vi "Read Refrigerant File_d.vi"(6 "error in (no error)":errorcluster, 7 "Clear Memory":bool, 8 "Refprop Main Directory":path, 9 "Refrigerant File":string) -> (0 "error out":errorcluster, 2 "Mixure Cluster":T1)   [LabVIEW 2017]
doc: "Developed by:\nGreg Sussman\nProcess Automation Corp\nwww.processauto.com\n(267)685-1249"
uses:
  Mixture Composition cluster_d.ctl
panel:
  out "memory counter":i32
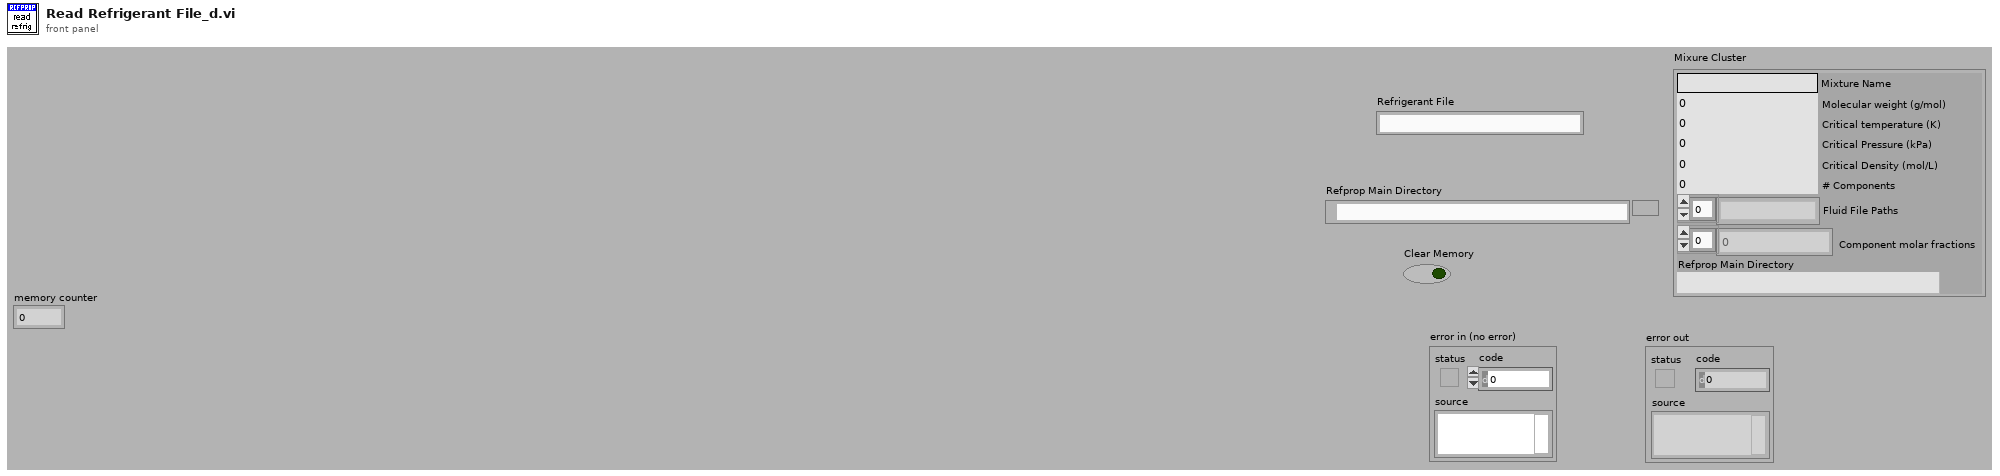
[diagram p1: front panel]
types:
  T1 = typedef "Mixture Composition cluster_d.ctl" = cluster{"Mixture Name":string, "Molecular weight (g/mol)":dbl, "Critical temperature (K)":dbl, "Critical Pressure (kPa)":dbl, "Critical Density (mol/L)":dbl, "# Components":i32, "Fluid File Paths":path[], "Component molar fractions":dbl[], "Refprop Main Directory":path}
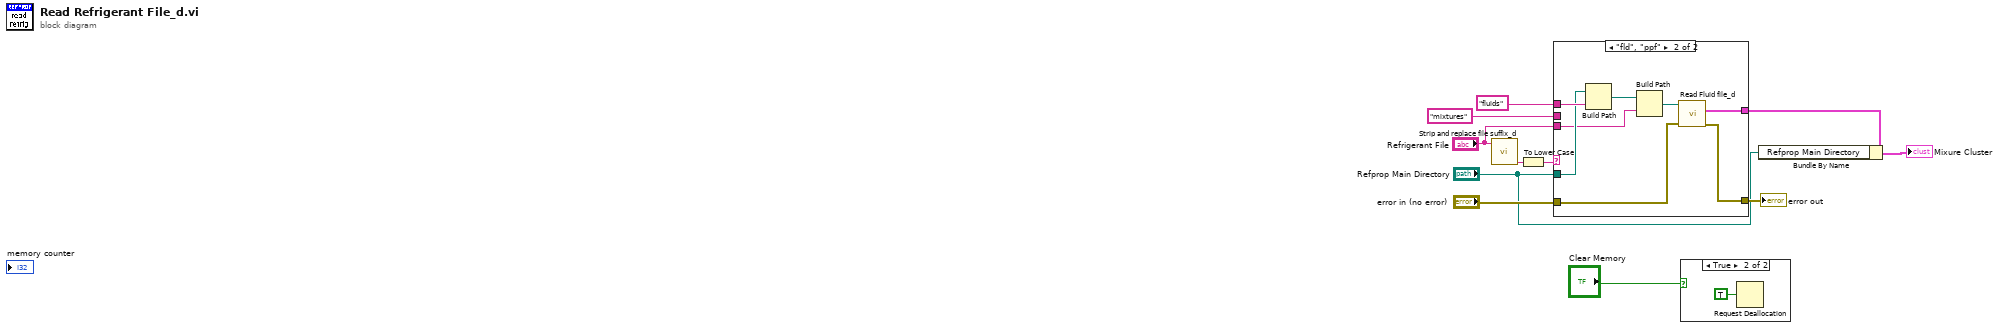
[diagram p0: block diagram]
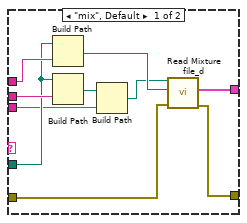
[diagram p3: hidden frame]
diagram:
  n1 = call "Strip and replace file suffix_d.vi"("File Name"="Refrigerant File") -> ("Old File Suffix OUT"=w8:string)  [unwired: 3 in, 1 out]
  n2 = To Lower Case(string=w8) -> (all lower case string=w11:string)
  n3 = case shown="\"fld\", \"ppf\"" w11 {
    tunnel: "Refprop Main Directory" -> [w15 w25]
    tunnel: [w21 w29] -> w3
    tunnel: "error in (no error)" -> [w20 w28]
    tunnel: [w19 w27] -> w9
    tunnel: "fluids" -> [w16 w26]
    tunnel: "Refrigerant File" -> [w13 w23]
    tunnel: "mixtures" -> [w18 _]
    frame "mix", Default {
      n4 = Build Path(base path=w15, name or relative path=w16) -> (appended path=w14:path)
      n5 = Build Path(base path=w15, name or relative path=w18) -> (appended path=w17:path)
      n6 = Build Path(base path=w17, name or relative path=w13) -> (appended path=w12:path)
      n7 = call "Read Mixture file_d.vi"("error in (no error)"=w20, "Dir containing fluid files"=w14, "Mixture File"=w12) -> ("error out"=w19:errorcluster, "Mixure Cluster"=w21:T1)  [unwired: 5 in]
    }
    frame "fld", "ppf" {
      n8 = Build Path(base path=w25, name or relative path=w26) -> (appended path=w24:path)
      n9 = Build Path(base path=w24, name or relative path=w23) -> (appended path=w22:path)
      n10 = call "Read Fluid file_d.vi"("error in (no error)"=w28, "Fluid File"=w22) -> ("error out"=w27:errorcluster, "Fluid Cluster"=w29:T1)  [unwired: 6 in]
    }
  }
  "error out" <- w9
  n11 = case shown="True" "Clear Memory" {
    frame False {
    }
    frame True {
      n12 = Request Deallocation(TRUE ("标志")) -> ()
    }
  }
  n13 = Bundle By Name(cluster=w3, "Refprop Main Directory"="Refprop Main Directory") -> (→"Mixure Cluster":T1)
